vi "总磷总氮通讯.vi"() -> ()   [LabVIEW 2016, in "斯坦道总氮.lvlib"]
uses:
  <vilib>/NI/Modbus Library/API/Wrapper/Create TCP Slave.vi
  <vilib>/Utility/config.llb/Write Key (Boolean).vi
  <vilib>/Utility/config.llb/Write Key (String).vi
  <vilib>/Plasmionique/MB Master/MB_Master/MB_Master.lvclass
  <vilib>/NI/Modbus Library/API/Slave/Modbus Slave.lvclass
  <vilib>/Utility/config.llb/NI_LVConfig.lvlib
  <vilib>/Plasmionique/MB Master/MB Master.lvlib
  <vilib>/NI/Modbus Library/API/Wrapper/API Main.lvlib
panel:
  out "氨氮状态告警区":u16[](array[numeric])
  out "氨氮测量数据区":u16[](array[numeric])
  out "COD测量数据区":u16[](array[numeric])
  out "COD状态告警区":u16[](array[numeric])
  out "总氮测量数据区":u16[](array[numeric])
  out "总氮状态告警区":u16[](array[numeric])
  out "总磷状态告警区":u16[](array[numeric])
  out "总磷测量数据区":u16[](array[numeric])
  out "序列号":string
  out "状态告警区":T1 {"告警代码" items=["无告警", "缺试剂告警", "缺水样告警", "缺蒸馏水告警", "缺标液告警", "仪表漏液告警", "标定异常告警", "超量程告警", "加热异常", "低试剂预警", "超上限告警", "超下限告警", "仪表内部其他异常", "滴定异常告警", "电极异常告警", "量程切换告警", "参数设置告警", "PH电极电位异常", "电导率电极异常", "浊度光度异常", "溶解氧电极异常", "溶解氧光强异常", "温度异常告警", "PH异常告警", "溶解氧异常告警", "电导率异常告警", "浊度异常告警", "叶绿素异常告警", "藻密度异常告警", "蓝绿藻异常告警", "ORP异常告警", "氨氮异常告警", "清洁刷异常告警", "SD卡异常告警", "蓝牙异常告警", "Wifi异常告警", "流程异常告警"]; "故障代码" items=["无故障", "电机故障", "温度故障", "通讯故障", "滴定故障"]}
  out "测量数据区":T2 {"单位" items=["ug/L", "mg/L", "ppm", "mg/m3", "cm", "ppb", "ug/m3", "%", "nmol/mol", "umol/mol", "MPN/L", "MPN/100ml", "ng/m3", "NTU", "无量纲", "ms/cm", "us/cm", "℃", "mV", "万个/L"]}
  out "status":bool
  out "关键参数区":T3
  in  "读关键参数区":bool
  in  "读状态告警区":bool
  in  "读测量数据区":bool
  in  "站号":u16(ring) items=["总磷"=1, "氨氮"=3]
  in  "停止":bool
  in  "启动":bool
  in  "控制命令":u16(ring) items=["启动测量"=1, "标样核查"=2, "零点核查"=3, "跨度核查"=4, "空白测试"=5, "平行样测试"=6, "加标回收"=7, "空白校准"=8, "标样校准"=9, "初始化（清洗）"=10, "停止测试"=11, "仪器重启"=12, "校时"=13, "模式设置"=14, "测量间隔设置"=15]
  in  "控制命令参数":u16[](array[numeric]) format="%04xH"
  in  "VISA Resource":refnum<visa-resource-name>
  in  "启用模块":bool
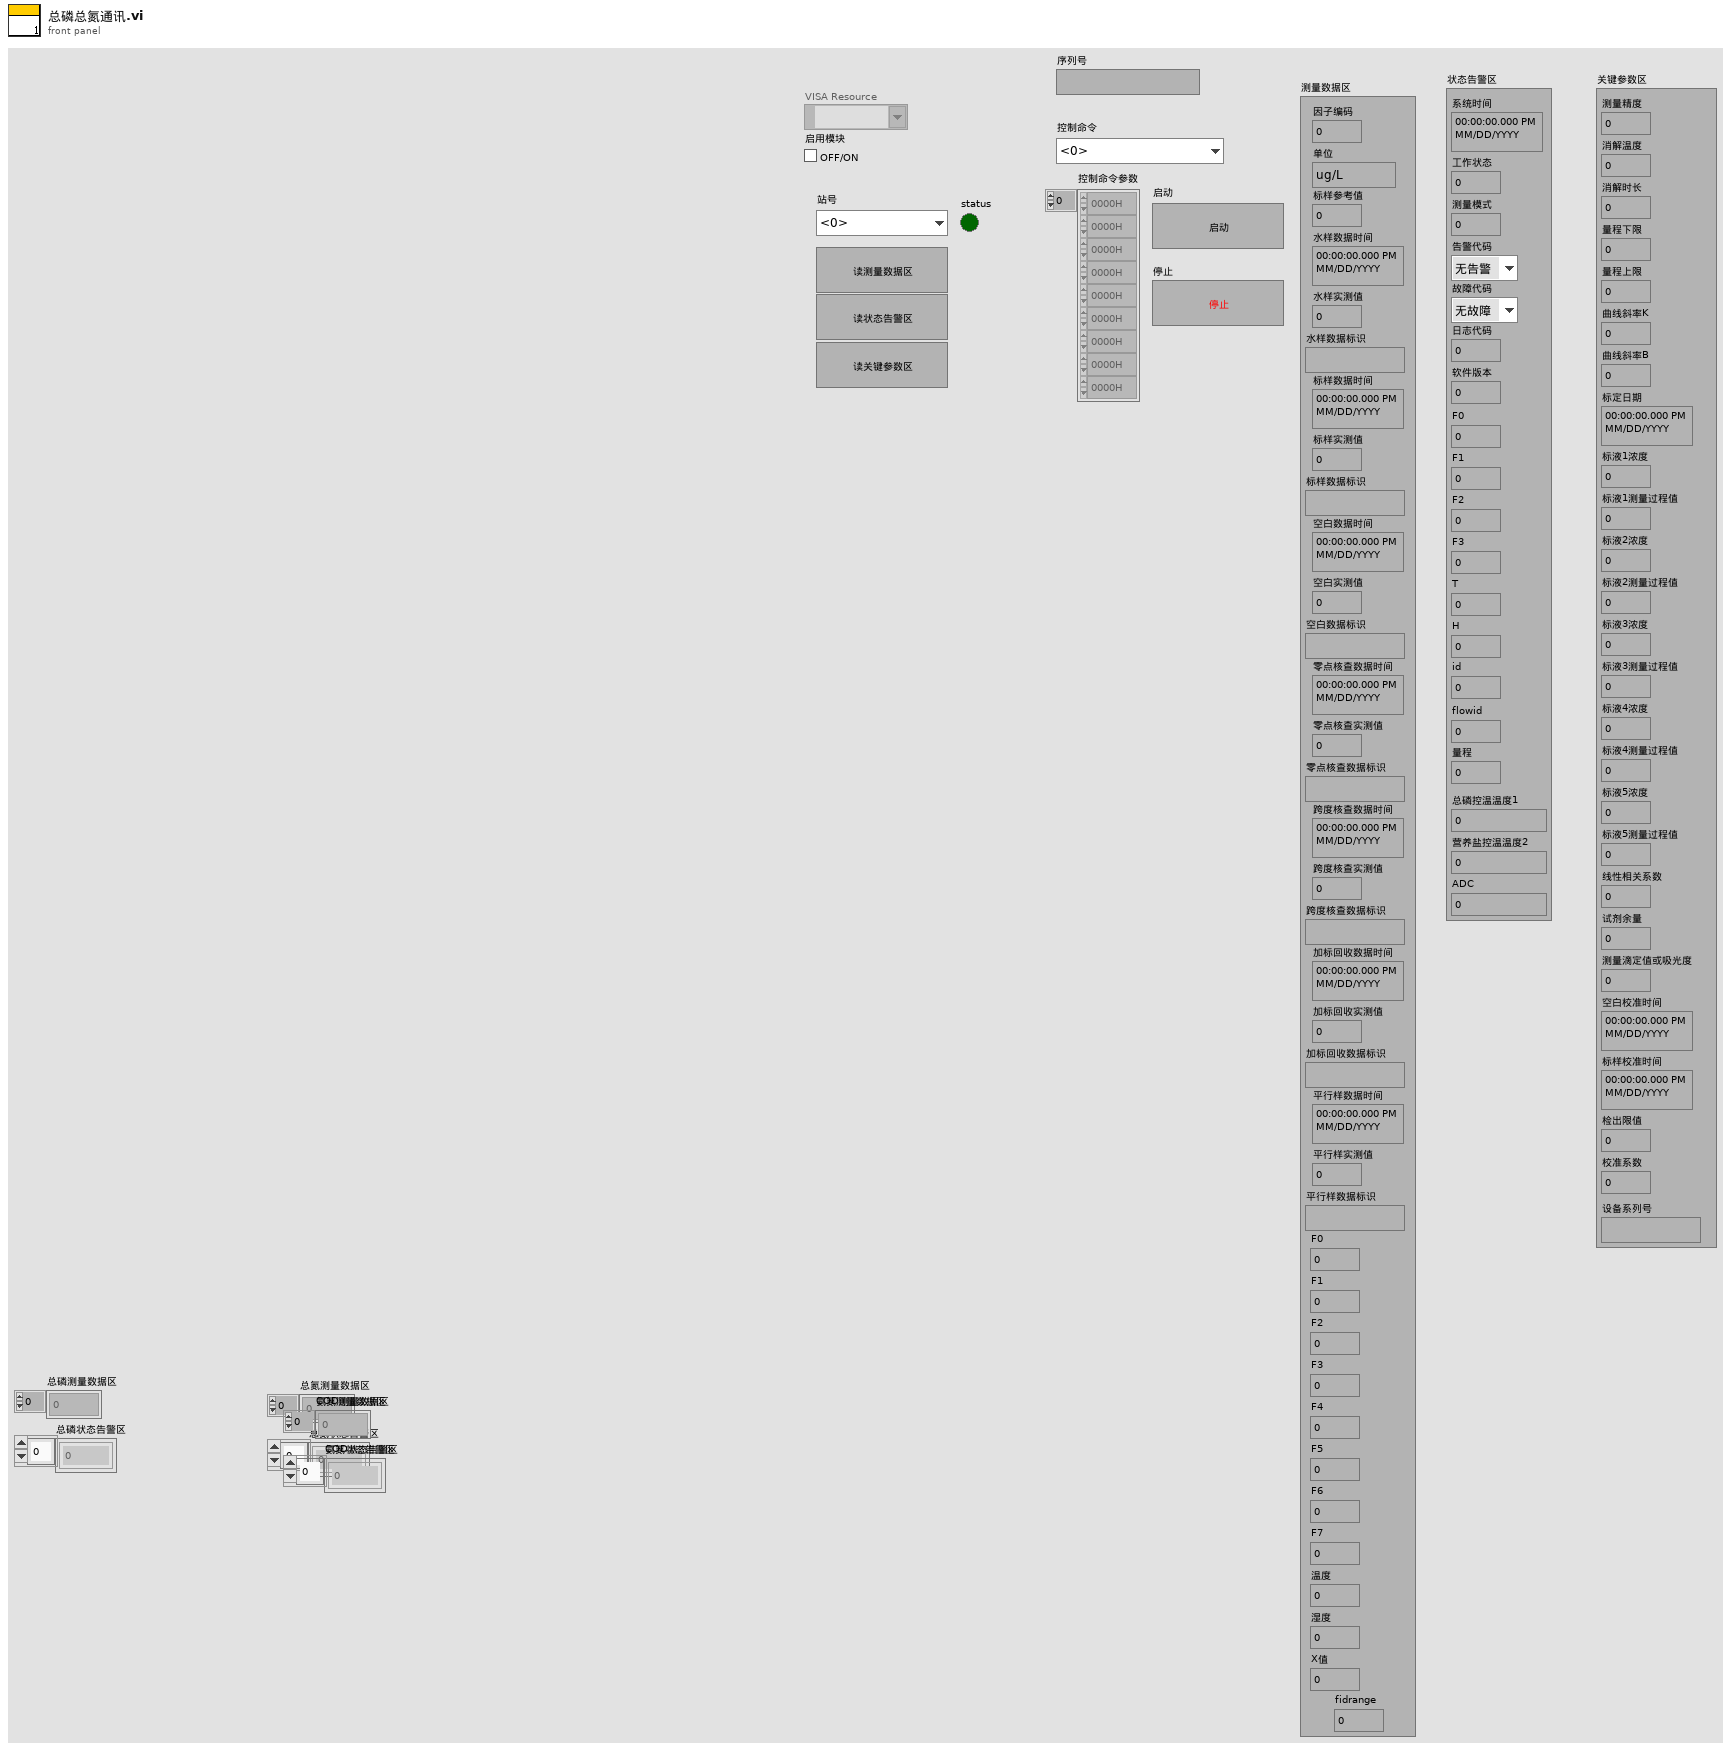
[diagram p1: front panel]
types:
  T1 = cluster{"系统时间":timestamp, "工作状态":u16, "测量模式":u16, "告警代码":u16, "故障代码":u16, "日志代码":u16, "软件版本":u16, "F0":sgl, "F1":sgl, "F2":sgl, "F3":sgl, "T":sgl, "H":sgl, "id":u16, "flowid":u16, "量程":u16, "总磷控温温度1":sgl, "营养盐控温温度2":sgl, "ADC":sgl}
  T2 = cluster{"因子编码":u32, "单位":u16, "标样参考值":sgl, "水样数据时间":timestamp, "水样实测值":sgl, "水样数据标识":string, "标样数据时间":timestamp, "标样实测值":sgl, "标样数据标识":string, "空白数据时间":timestamp, "空白实测值":sgl, "空白数据标识":string, "零点核查数据时间":timestamp, "零点核查实测值":sgl, "零点核查数据标识":string, "跨度核查数据时间":timestamp, "跨度核查实测值":sgl, "跨度核查数据标识":string, "加标回收数据时间":timestamp, "加标回收实测值":sgl, "加标回收数据标识":string, "平行样数据时间":timestamp, "平行样实测值":sgl, "平行样数据标识":string, "F0":sgl, "F1":sgl, "F2":sgl, "F3":sgl, "F4":sgl, "F5":sgl, "F6":sgl, "F7":sgl, "温度":sgl, "湿度":sgl, "X值":sgl, "fidrange":u16}
  T3 = cluster{"测量精度":u16, "消解温度":u16, "消解时长":u16, "量程下限":sgl, "量程上限":sgl, "曲线斜率K":sgl, "曲线斜率B":sgl, "标定日期":timestamp, "标液1浓度":sgl, "标液1测量过程值":sgl, "标液2浓度":sgl, "标液2测量过程值":sgl, "标液3浓度":sgl, "标液3测量过程值":sgl, "标液4浓度":sgl, "标液4测量过程值":sgl, "标液5浓度":sgl, "标液5测量过程值":sgl, "线性相关系数":sgl, "试剂余量":u32, "测量滴定值或吸光度":sgl, "空白校准时间":timestamp, "标样校准时间":timestamp, "检出限值":sgl, "校准系数":sgl, "设备系列号":string}
  T4 = cluster{"COD":bool, "氨氮":bool, "总氮":bool, "总磷":bool}
  T5 = typedef "NI_LVConfig.lvlib/Config Data RefNum.ctl" = refnum<k1>
  T6 = enum8{"Enabled", "Disabled", "Disabled and Grayed Out"}
  T7 = cluster{"系统时间":timestamp, "工作状态":enum16{"空闲", "水样测试", "标样核查", "零点核查", "跨度核查", "空白测试", "平行样测试", "加标回收", "空白校准", "标样校准", "初始化（清洗）"}, "测量模式":enum16{"待机", "连续模式", "周期模式", "定点模式", "受控模式", "手动模式"}, "告警代码":u16, "故障代码":u16, "日志代码":u16, "软件版本":u16, "F0":sgl, "F1":sgl, "F2":sgl, "F3":sgl, "T":sgl, "H":sgl, "id":u16, "flowid":u16, "量程":u16, "总磷控温温度1":sgl, "营养盐控温温度2":sgl, "ADC":sgl}
  T8 = cluster{"水样测试量程模式":enum16{"H", "L", "AUTO"}, "空白核查量程模式":enum16{"H", "L", "AUTO"}, "跨度核查量程模式":enum16{"H", "L", "AUTO"}, "加标回收量程模式":enum16{"H", "L", "AUTO"}}
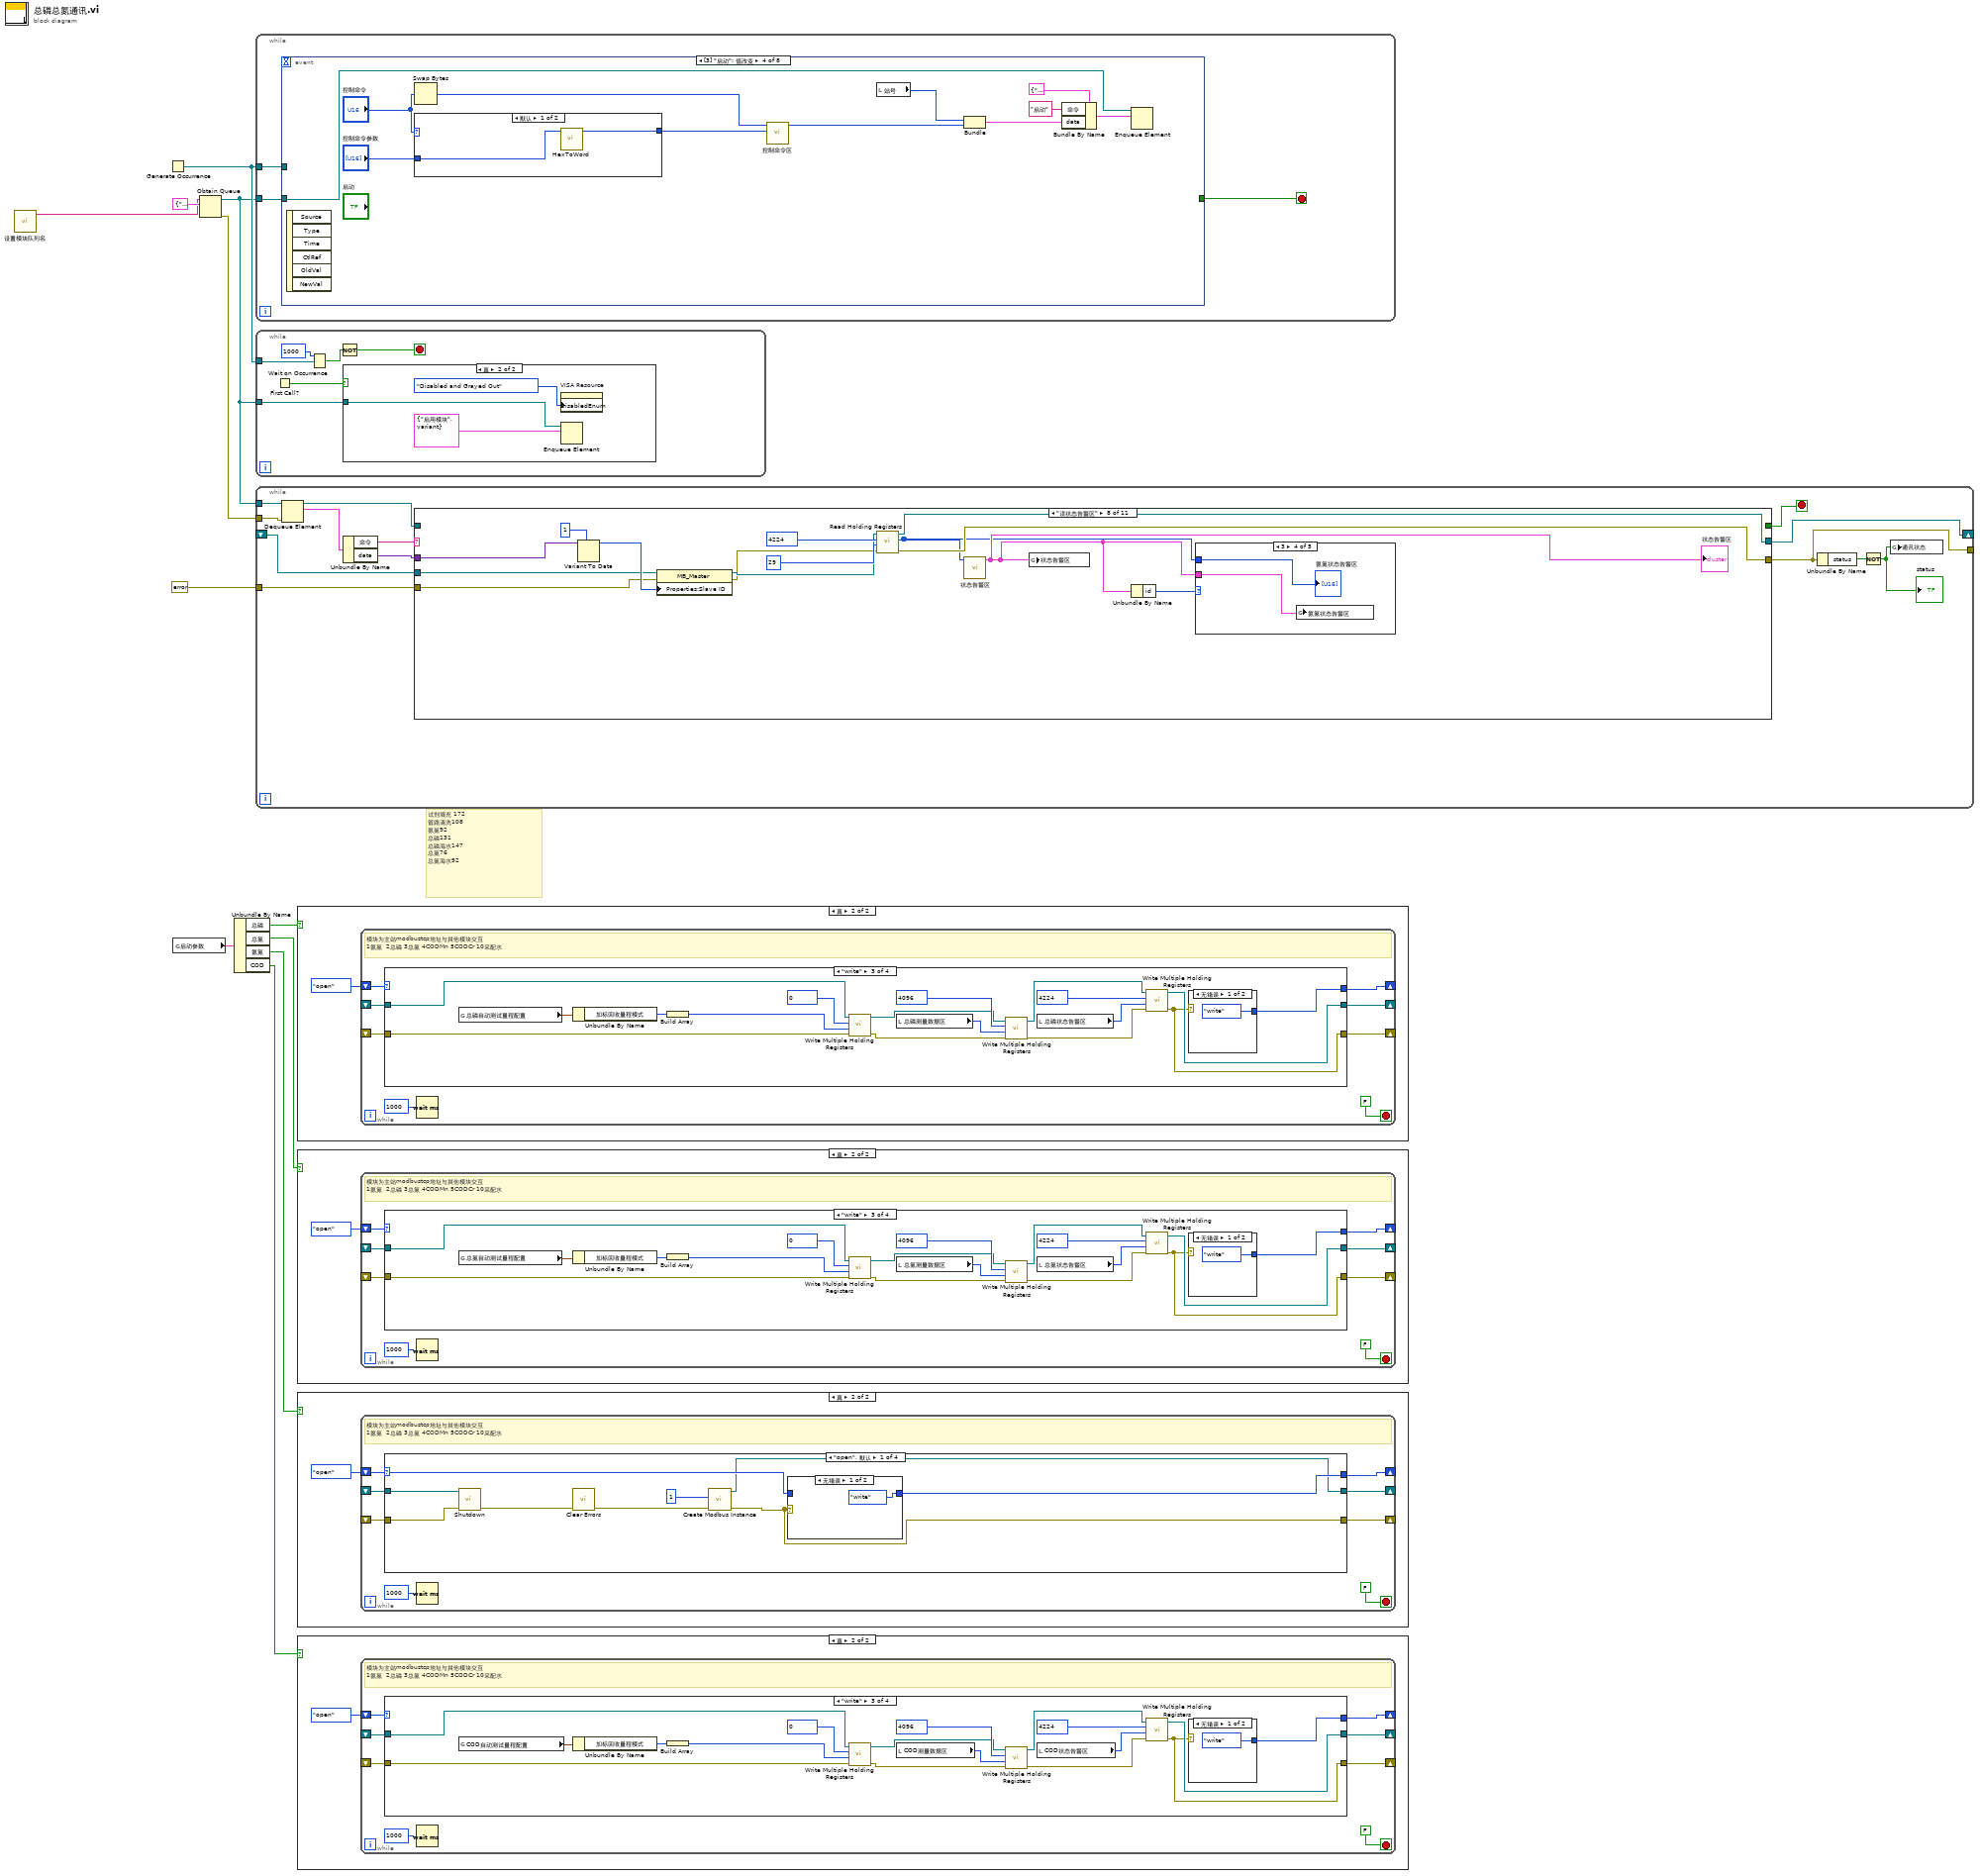
[diagram p0: block diagram]
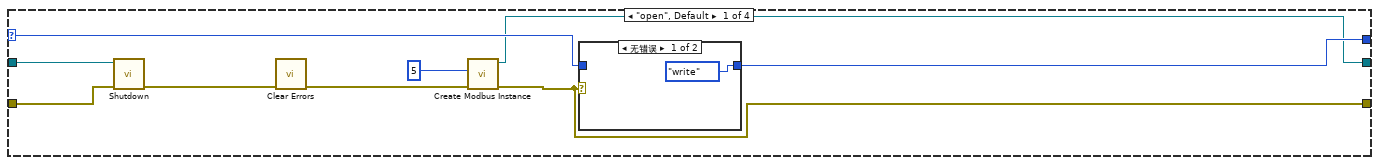
[diagram p3: hidden frame]
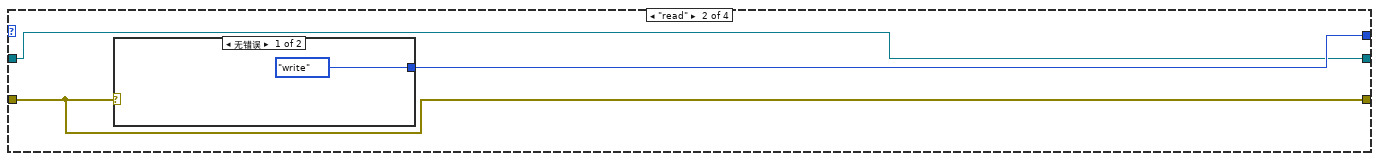
[diagram p5: hidden frame]
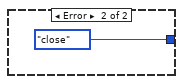
[diagram p6: hidden frame]
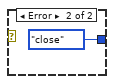
[diagram p7: hidden frame]
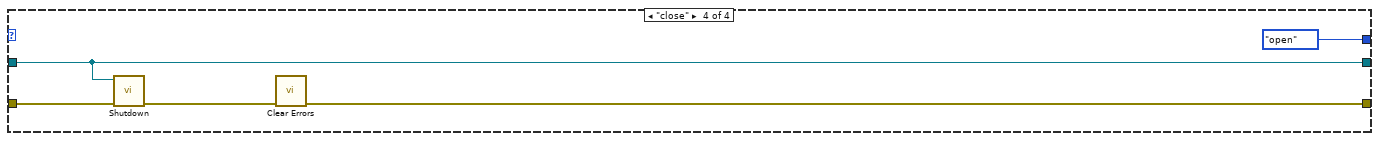
[diagram p8: hidden frame]
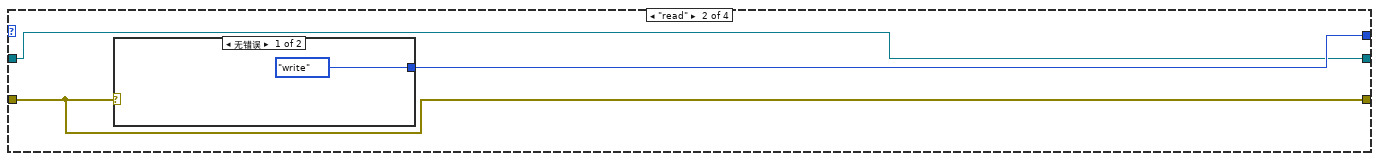
[diagram p11: hidden frame]
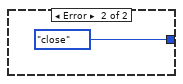
[diagram p12: hidden frame]
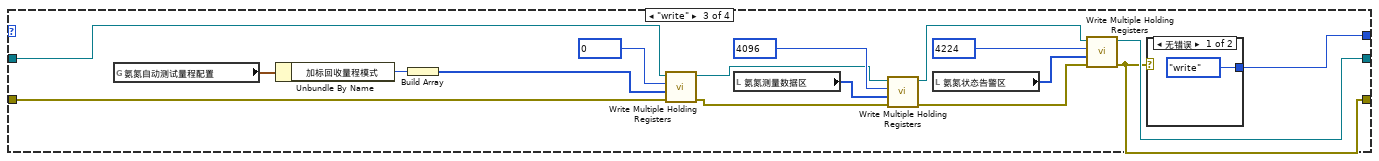
[diagram p13: hidden frame]
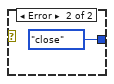
[diagram p14: hidden frame]
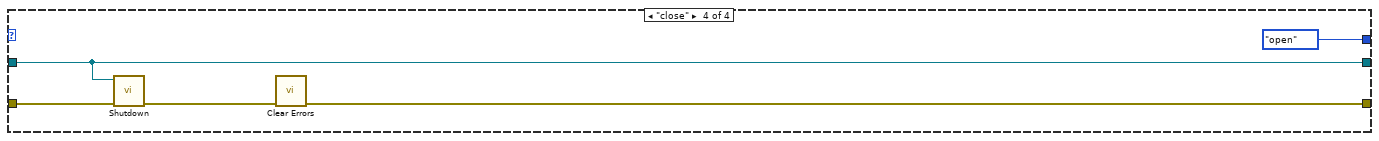
[diagram p15: hidden frame]
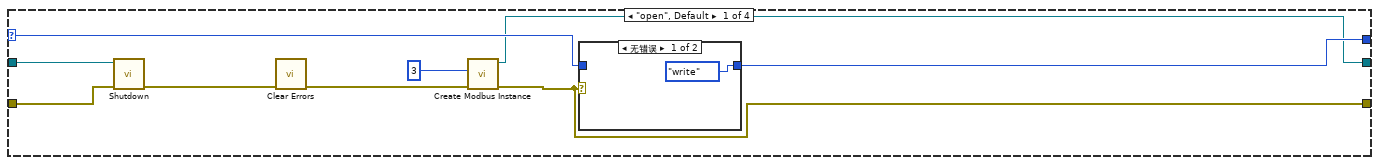
[diagram p17: hidden frame]
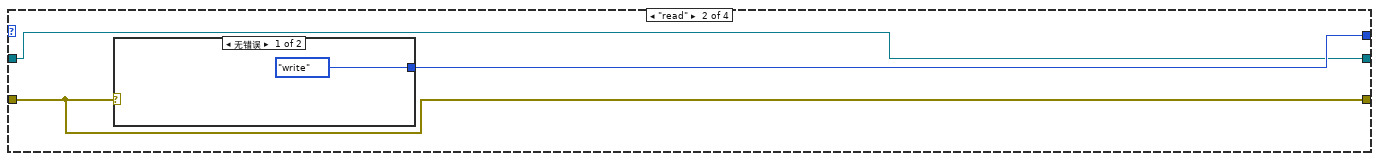
[diagram p19: hidden frame]
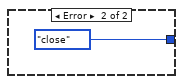
[diagram p20: hidden frame]
diagram:
  # "试剂填充 172 \n管路清洗108\n氨氮92\n总磷131\n总磷海水147\n总氮76\n总氮海水92"
  n1 = call "设置模块队列名.vi"() -> ("Msg"=w1:string)  [unwired: 5 in]
  n2 = Generate Occurrence() -> (w8:refnum<k4>)
  n3 = global read "总磷总氮断电保存全局变量.vi" "启动参数"() -> (w6:T4)
  n4 = Obtain Queue(name (unnamed)=w1, element data type=cluster{"命令":string, "data":variant} {"命令"="", "data"=variant}) -> (queue out=w7:refnum<queue>, error out=w10:errorcluster)  [unwired: 3 in, 1 out]
  n5 = Unbundle By Name(w6) -> ("总磷"=w5:bool, "总氮"=w4:bool, "氨氮"=w3:bool, "COD"=w2:bool)
  n6 = while {
    tunnel: w7 -> [w14]
    tunnel: w8 -> [w12]
    stop <- w13 stop-if-true
    n7 = event shown="[3] \"启动\": 值改变" {
      selector: _ -> [_ _ _ _ _ _ _ _]
      dyn-events: _ -> [_ _ _ _ _ _ _ _]
      timeout: _ -> [_ _ _ _ _ _ _ _]
      tunnel: w14 -> [_ _ _ w45 w52 w58 w63 w68]
      tunnel: [_ _ _ _ "停止" _ _ _] -> w13
      tunnel: w12 -> [_ _ _ _ w49 _ _ _]
      event Timeout {
        n8 = event-data() -> ()  [unwired: 1 in, 3 out]
      }
      event "启用模块": Value Change {
        n9 = event-data() -> ("NewVal"=w15:bool)  [unwired: 1 in, 5 out]
        n10 = call <vilib>:"Application Directory.vi"() -> ("Application Directory"=w17:path)
        n11 = Build Path(base path=w17, name or relative path="data\\set.ini" ("名称或相对路径")) -> (appended path=w18:path)
        n12 = call <vilib>:"Open Config Data.vi"("configuration file path"=w18) -> ("error out"=w24:errorcluster, "refnum"=w23:T5)  [unwired: 8 in, 1 out]
        n13 = call-poly <vilib>:"Write Key.vi"("section"="总磷总氮", "error in (no error)"=w24, "value"=w15, "key"="模块启用", "refnum"=w23) -> ("error out"=w20:errorcluster, "refnum out"=w16:T5)  [unwired: 4 in, 1 out]
        n14 = call <vilib>:"Close Config Data.vi"("error in (no error)"=w20, "refnum"=w16) -> ()  [unwired: 8 in, 2 out]
      }
      event "VISA Resource": Value Change {
        n15 = event-data() -> ()  [unwired: 1 in, 6 out]
        n16 = call <vilib>:"Application Directory.vi"() -> ("Application Directory"=w27:path)
        n17 = Build Path(base path=w27, name or relative path="data\\set.ini" ("名称或相对路径")) -> (appended path=w28:path)
        n18 = call <vilib>:"Open Config Data.vi"("configuration file path"=w28) -> ("error out"=w34:errorcluster, "refnum"=w33:T5)  [unwired: 8 in, 1 out]
        n19 = call-poly <vilib>:"Write Key.vi"("section"="总磷总氮", "error in (no error)"=w34, "value"="VISA Resource", "key"="串口", "refnum"=w33) -> ("error out"=w30:errorcluster, "refnum out"=w26:T5)  [unwired: 4 in, 1 out]
        n20 = call <vilib>:"Close Config Data.vi"("error in (no error)"=w30, "refnum"=w26) -> ()  [unwired: 8 in, 2 out]
      }
      event "启动": Value Change {
        n21 = event-data() -> ()  [unwired: 1 in, 6 out]
        n22 = Swap Bytes(anything="控制命令") -> (byte swapped=w38:u16)
        n23 = case shown="默认" "控制命令" {
          tunnel: "控制命令参数" -> [w47 w48]
          tunnel: [w46 w48] -> w35
          frame Default {
            n24 = call "HexToWord.vi"("数组"=w47) -> ("WORD"=w46:u16[])  [unwired: 10 in]
          }
          frame 13 {
          }
        }
        n25 = call "控制命令区.vi"("控制命令参数"=w35, "控制命令"=w38) -> ("控制命令"=w41:u16[])  [unwired: 9 in]
        n26 = local read "站号"() -> (w40:u16)
        n27 = Bundle("站号"=w40, "控制命令"=w41) -> (w39:cluster{"站号":u16, "控制命令":u16[]})  [unwired: 1 in]
        n28 = Bundle By Name(cluster=cluster{"命令":string, "data":variant} {"命令"="", "data"=variant} ("元素"), "命令"="启动", "data"=w39) -> (w43:cluster{"命令":string, "data":variant})
        n29 = Enqueue Element(queue=w45, element=w43) -> ()  [unwired: 2 in, 3 out]
      }
      event "停止": Value Change {
        n30 = event-data() -> ()  [unwired: 1 in, 6 out]
        n31 = Set Occurrence(w49) -> ()
        n32 = Flush Queue(queue=w52) -> (queue out=w51:refnum<queue>)  [unwired: 1 in, 2 out]
        n33 = Enqueue Element(queue=w51, element=cluster{"命令":string, "data":variant} {"命令"="shutdown", "data"=variant} ("元素")) -> ()  [unwired: 2 in, 3 out]
      }
      event "读测量数据区": Value Change {
        n34 = event-data() -> ()  [unwired: 1 in, 6 out]
        n35 = Bundle By Name(cluster=cluster{"命令":string, "data":variant} {"命令"="", "data"=variant} ("元素"), "命令"="读测量数据区", "data"="站号") -> (w56:cluster{"命令":string, "data":variant})
        n36 = Enqueue Element(queue=w58, element=w56) -> ()  [unwired: 2 in, 3 out]
      }
      event "读状态告警区": Value Change {
        n37 = event-data() -> ()  [unwired: 1 in, 6 out]
        n38 = local read "站号"() -> (w59:u16)
        n39 = Bundle By Name(cluster=cluster{"命令":string, "data":variant} {"命令"="", "data"=variant} ("元素"), "命令"="读状态告警区", "data"=w59) -> (w61:cluster{"命令":string, "data":variant})
        n40 = Enqueue Element(queue=w63, element=w61) -> ()  [unwired: 2 in, 3 out]
      }
      event "读关键参数区": Value Change {
        n41 = event-data() -> ()  [unwired: 1 in, 6 out]
        n42 = local read "站号"() -> (w64:u16)
        n43 = Bundle By Name(cluster=cluster{"命令":string, "data":variant} {"命令"="", "data"=variant} ("元素"), "命令"="读关键参数区", "data"=w64) -> (w66:cluster{"命令":string, "data":variant})
        n44 = Enqueue Element(queue=w68, element=w66) -> ()  [unwired: 2 in, 3 out]
      }
    }
  }
  n45 = while {
    tunnel: w8 -> [w74]
    tunnel: w7 -> [w70]
    stop <- w71 stop-if-true
    n46 = First Call?() -> (First Call?: T/F=w69:bool)
    n47 = Wait on Occurrence(2:w74, 3:1000 ("毫秒超时(-1)")) -> (0:w72:bool)  [unwired: 1 in]
    n48 = Not(x=w72) -> (.not. x?=w71:bool)
    n49 = case shown="真" w69 {
      tunnel: w70 -> [_ w76]
      frame False {
      }
      frame True {
        n50 = property on="VISA Resource" class="VISAName"("DisabledEnum"=T6."Disabled and Grayed Out" ("禁用")) -> ()  [unwired: 2 in, 2 out]
        n51 = Enqueue Element(queue=w76, element=cluster{"命令":string, "data":variant} {"命令"="启用模块", "data"=variant} ("元素")) -> ()  [unwired: 2 in, 3 out]
      }
    }
  }
  n52 = while {
    tunnel: w7 -> [w90]
    tunnel: w10 -> [w89]
    shift-right: [w87] -> _
    shift-left: _ -> [w86]
    tunnel: errorcluster {"status"=FALSE, "code"=0, "source"=""} ("error out") -> [w85]
    tunnel: [w80] -> _
    stop <- w88 stop-if-true
    n53 = Dequeue Element(queue=w90, error in (no error)=w89) -> (queue out=w81:refnum<queue>, element=w83:cluster{"命令":string, "data":variant})  [unwired: 1 in, 2 out]
    n54 = Unbundle By Name(w83) -> ("命令"=w84:string, "data"=w82:variant)
    n55 = case shown="\"读状态告警区\"" w84 {
      tunnel: w82 -> [_ _ _ w109 w120 w137 w147 w173 w195 w209 _]
      tunnel: w81 -> [_ _ _ _ _ _ _ _ _ _ w222]
      tunnel: [_ _ _ _ _ _ _ _ _ _ TRUE] -> w88
      tunnel: [w91 w93 w96 w112 w123 w139 w151 w182 w202 w216 w218] -> w87
      tunnel: [w92 w94 w97 w111 w122 w138 w152 w172 w203 w217 w219] -> w80
      tunnel: w86 -> [w91 _ w96 w108 w119 w136 w146 w176 w198 w212 w218]
      tunnel: w85 -> [w92 _ w99 w105 w116 w133 w144 w177 w199 w213 w220]
      frame Default {
      }
      frame "启用模块" {
        n56 = call "总磷总氮MB_api.vi"("STEP"=enum16{"open", "read", "write", "close"}."open") -> ("error out"=w94:errorcluster, "MB session out"=w93:refnum<class "MB_Master.lvclass">)  [unwired: 8 in, 1 out]
        n57 = global write "VAR总磷总氮全局变量.vi" "MB session in"(w93) -> ()
      }
      frame "停用模块" {
        n58 = call-dynamic "Close Session.vi"("error in (no error)"=w99, "MB session in"=w96) -> ("error out"=w98:errorcluster)  [unwired: 9 in]
        n59 = call <vilib>:"Clear Errors.vi"("error in (no error)"=w98) -> ("error out"=w97:errorcluster)  [unwired: 5 in, 1 out]
      }
      frame "启动" {
        n60 = Variant To Data(type=cluster{"站号":u16, "控制命令":u16[]} {"站号"=0, "控制命令"=[]} ("输出簇"), Variant=w109) -> (data=w103:cluster{"站号":u16, "控制命令":u16[]})  [unwired: 1 in, 1 out]
        n61 = Unbundle By Name(w103) -> ("站号"=w102:u16, "控制命令"=w100:u16[])
        n62 = Index Array(array=w100) -> (element=w101:u16)  [unwired: 1 in]
        n63 = property class="MB_Master"(reference=w108, error in=w105, "Properties:Slave ID"=w102) -> (reference out=w107:refnum<class "MB_Master.lvclass">, error out=w106:errorcluster)
        n64 = global write "VAR总磷总氮全局变量.vi" "控制命令"(w101) -> ()
        n65 = call <vilib>:"Write Multiple Registers.vi"("error in (no error)"=w106, "values"=w100, "starting address"=u16 4608, "MB session in"=w107) -> ("error out"=w111:errorcluster, "MB session out"=w112:refnum<class "MB_Master.lvclass">)  [unwired: 6 in]
      }
      frame "盲样测试" {
        n66 = Variant To Data(type=0, Variant=w120) -> (data=w113:i32)  [unwired: 1 in, 1 out]
        n67 = case shown="默认" w113 {
          tunnel: [u16[] [] ("values") u16[] [33539, 0] ("values") u16[] [23555, 0] ("values")] -> w115
          frame Default {
          }
          frame 1 {
            # "总磷盲样测试命令"
          }
          frame 3 {
            # "氨氮盲样测试"
          }
        }
        n68 = property class="MB_Master"(reference=w119, error in=w116, "Properties:Slave ID"=w113) -> (reference out=w118:refnum<class "MB_Master.lvclass">, error out=w117:errorcluster)
        n69 = call <vilib>:"Write Multiple Registers.vi"("error in (no error)"=w117, "values"=w115, "starting address"=u16 24592, "MB session in"=w118) -> ("error out"=w122:errorcluster, "MB session out"=w123:refnum<class "MB_Master.lvclass">)  [unwired: 6 in]
      }
      frame "debug" {
        n70 = Variant To Data(type=cluster{"站号":u16, "控制命令":u16[]} {"站号"=0, "控制命令"=[]} ("输出簇"), Variant=w137) -> (data=w131:cluster{"站号":u16, "控制命令":u16[]})  [unwired: 1 in, 1 out]
        n71 = Unbundle By Name(w131) -> ("站号"=w130:u16, "控制命令"=w128:u16[])
        n72 = Index Array(array=w128) -> (element=w129:u16)  [unwired: 1 in]
        n73 = property class="MB_Master"(reference=w136, error in=w133, "Properties:Slave ID"=w130) -> (reference out=w135:refnum<class "MB_Master.lvclass">, error out=w134:errorcluster)
        n74 = global write "VAR总磷总氮全局变量.vi" "控制命令"(w129) -> ()
        n75 = call <vilib>:"Write Multiple Registers.vi"("error in (no error)"=w134, "values"=w128, "starting address"=u16 24594, "MB session in"=w135) -> ("error out"=w138:errorcluster, "MB session out"=w139:refnum<class "MB_Master.lvclass">)  [unwired: 6 in]
      }
      frame "读测量数据区" {
        n76 = Variant To Data(type=u8 1 ("Slave ID"), Variant=w147) -> (data=w142:u8)  [unwired: 1 in, 1 out]
        n77 = property class="MB_Master"(reference=w146, error in=w144, "Properties:Slave ID"=w142) -> (reference out=w145:refnum<class "MB_Master.lvclass">, error out=w143:errorcluster)
        n78 = call <vilib>:"Read Holding Registers.vi"("error in (no error)"=w143, "quantity"=u16 105, "starting address"=u16 4096, "MB session in"=w145) -> ("error out"=w152:errorcluster, "Registers"=w140:u16[], "MB session out"=w151:refnum<class "MB_Master.lvclass">)  [unwired: 5 in]
        n79 = call "测量数据区.vi"("数组"=w140) -> ("测量数据区"=w141:T2)  [unwired: 10 in]
        "测量数据区" <- w141
        n80 = global write "VAR总磷总氮全局变量.vi" "测量数据区"(w141) -> ()
        n81 = case shown="3" w142 {
          tunnel: w141 -> [_ w155 w164 w166 w168]
          tunnel: w140 -> [_ w156 w163 w165 w167]
          frame 0, Default {
          }
          frame 1 {
            n82 = global read "总磷总氮断电保存全局变量.vi" "启动参数"() -> (w154:T4)
            n83 = Unbundle By Name(w154) -> ("总氮"=w153:bool)
            n84 = case shown="真" w153 {
              tunnel: [w158 w161] -> w157
              tunnel: w155 -> [w158 w159]
              frame False {
              }
              frame True {
                # "启动总氮时间自动对齐"
                n85 = global read "VAR总磷总氮全局变量.vi" "总氮测量数据区"() -> (w162:T2)
                n86 = global read "VAR总磷总氮全局变量.vi" "总磷测量数据区"() -> (w160:T2)
                n87 = call "总磷数据时间处理.vi"("总磷修正数据输入"=w160, "总氮原始数据"=w162, "总磷原始数据"=w159) -> ("总磷修正数据输出"=w161:T2)  [unwired: 8 in]
              }
            }
            n88 = global write "VAR总磷总氮全局变量.vi" "总磷测量数据区"(w157) -> ()
            "总磷测量数据区" <- w156
          }
          frame 2 {
            n89 = global write "VAR总磷总氮全局变量.vi" "总氮测量数据区"(w164) -> ()
            "总氮测量数据区" <- w163
          }
          frame 3 {
            n90 = global write "VAR总磷总氮全局变量.vi" "氨氮测量数据区"(w166) -> ()
            "氨氮测量数据区" <- w165
          }
          frame 22 {
            n91 = global write "VAR总磷总氮全局变量.vi" "COD测量数据区"(w168) -> ()
            "COD测量数据区" <- w167
          }
        }
      }
      frame "读状态告警区" {
        n92 = Variant To Data(type=u8 1 ("Slave ID"), Variant=w173) -> (data=w178:u8)  [unwired: 1 in, 1 out]
        n93 = property class="MB_Master"(reference=w176, error in=w177, "Properties:Slave ID"=w178) -> (reference out=w175:refnum<class "MB_Master.lvclass">, error out=w174:errorcluster)
        n94 = call <vilib>:"Read Holding Registers.vi"("error in (no error)"=w174, "quantity"=u16 29, "starting address"=u16 4224, "MB session in"=w175) -> ("error out"=w172:errorcluster, "Registers"=w169:u16[], "MB session out"=w182:refnum<class "MB_Master.lvclass">)  [unwired: 5 in]
        n95 = call "状态告警区.vi"("数组"=w169) -> ("状态告警区"=w170:T7)  [unwired: 10 in]
        "状态告警区" <- w170
        n96 = global write "VAR总磷总氮全局变量.vi" "状态告警区"(w170) -> ()
        n97 = Unbundle By Name(w170) -> ("id"=w171:u16)
        n98 = case shown="3" w171 {
          tunnel: w170 -> [_ w184 w186 w188 w190]
          tunnel: w169 -> [_ w183 w185 w187 w189]
          frame 0, Default {
          }
          frame 1, 131 {
            n99 = global write "VAR总磷总氮全局变量.vi" "总磷状态告警区"(w184) -> ()
            "总磷状态告警区" <- w183
          }
          frame 2, 76 {
            n100 = global write "VAR总磷总氮全局变量.vi" "总氮状态告警区"(w186) -> ()
            "总氮状态告警区" <- w185
          }
          frame 3 {
            n101 = global write "VAR总磷总氮全局变量.vi" "氨氮状态告警区"(w188) -> ()
            "氨氮状态告警区" <- w187
          }
          frame 22 {
            n102 = global write "VAR总磷总氮全局变量.vi" "COD状态告警区"(w190) -> ()
            "COD状态告警区" <- w189
          }
        }
      }
      frame "读关键参数区" {
        n103 = Variant To Data(type=u8 1 ("Slave ID"), Variant=w195) -> (data=w193:u8)  [unwired: 1 in, 1 out]
        n104 = property class="MB_Master"(reference=w198, error in=w199, "Properties:Slave ID"=w193) -> (reference out=w197:refnum<class "MB_Master.lvclass">, error out=w196:errorcluster)
        n105 = call <vilib>:"Read Holding Registers.vi"("error in (no error)"=w196, "quantity"=u16 19, "starting address"=u16 4256, "MB session in"=w197) -> ("error out"=w203:errorcluster, "Registers"=w192:u16[], "MB session out"=w202:refnum<class "MB_Master.lvclass">)  [unwired: 5 in]
        n106 = call "关键参数区.vi"("数组"=w192) -> ("关键参数区"=w191:T3)  [unwired: 10 in]
        "关键参数区" <- w191
        n107 = global write "VAR总磷总氮全局变量.vi" "关键参数区"(w191) -> ()
      }
      frame "读序列号" {
        n108 = Variant To Data(type=u8 1 ("Slave ID"), Variant=w209) -> (data=w207:u8)  [unwired: 1 in, 1 out]
        n109 = property class="MB_Master"(reference=w212, error in=w213, "Properties:Slave ID"=w207) -> (reference out=w211:refnum<class "MB_Master.lvclass">, error out=w210:errorcluster)
        n110 = call <vilib>:"Read Holding Registers.vi"("error in (no error)"=w210, "quantity"=u16 6, "starting address"=u16 4, "MB session in"=w211) -> ("error out"=w217:errorcluster, "Registers"=w206:u16[], "MB session out"=w216:refnum<class "MB_Master.lvclass">)  [unwired: 5 in]
        n111 = call "HexToString.vi"("数组"=w206) -> ("STRING"=w205:string[])  [unwired: 10 in]
        n112 = Index Array(array=w205) -> (element=w204:string)  [unwired: 1 in]
        "序列号" <- w204
        n113 = global write "VAR总磷总氮全局变量.vi" "序列号"(w204) -> ()
      }
      frame "shutdown" {
        n114 = Flush Queue(queue=w222) -> (queue out=w221:refnum<queue>)  [unwired: 1 in, 2 out]
        n115 = call-dynamic "Close Session.vi"("error in (no error)"=w220, "MB session in"=w218) -> ("error out"=w219:errorcluster)  [unwired: 9 in]
        n116 = Release Queue(queue=w221) -> ()  [unwired: 2 in, 3 out]
      }
    }
    n117 = Unbundle By Name(w80) -> ("status"=w79:bool)
    n118 = Not(x=w79) -> (.not. x?=w78:bool)
    "status" <- w78
    n119 = global write "VAR总磷总氮全局变量.vi" "通讯状态"(w78) -> ()
  }
  n120 = case shown="真" w5 {
    frame False {
    }
    frame True {
      n121 = while {
        shift-right: [w230] -> _
        shift-left: _ -> [w232]
        shift-right: [w229] -> _
        shift-left: _ -> [w231]
        shift-right: [w226] -> _
        shift-left: enum16{"open", "read", "write", "close"}."open" -> [w227]
        stop <- FALSE stop-if-true
        # "模块为主站modbustcp地址与其他模块交互\n1氨氮  2总磷 3总氮 4CODMn 5CODCr 10采配水"
        n122 = case shown="\"write\"" w227 {
          selector: w227 -> [w241 _ _ _]
          tunnel: w232 -> [w235 w244 w255 w270]
          tunnel: w231 -> [w234 w245 w251 w269]
          tunnel: [w238 w244 w261 w270] -> w230
          tunnel: [w237 w245 w260 w272] -> w229
          tunnel: [w240 w246 w265 enum16{"open", "read", "write", "close"}."open"] -> w226
          frame "open", Default {
            n123 = call-dynamic "Shutdown.vi"("error in"=w234, "Modbus slave in"=w235) -> ("error out"=w233:errorcluster)  [unwired: 9 in]
            n124 = call <vilib>:"Clear Errors.vi"("error in (no error)"=w233) -> ("error out"=w236:errorcluster)  [unwired: 5 in, 1 out]
            n125 = call-poly <vilib>:"Create Modbus Instance.vi"("error in"=w236, "port (502)"=u16 2) -> ("error out"=w237:errorcluster, "TCP slave instance"=w238:refnum<class "Modbus Slave.lvclass">)  [unwired: 8 in]
            n126 = case shown="无错误" w237 {
              tunnel: w241 -> [_ w243]
              tunnel: [enum16{"open", "read", "write", "close"}."write" w243] -> w240
              frame No Error {
              }
              frame Error {
              }
            }
          }
          frame "read" {
            n127 = case shown="无错误" w245 {
              tunnel: [enum16{"open", "read", "write", "close"}."write" enum16{"open", "read", "write", "close"}."close"] -> w246
              frame No Error {
              }
              frame Error {
              }
            }
          }
          frame "write" {
            n128 = global read "总磷总氮断电保存全局变量.vi" "总磷自动测试量程配置"() -> (w254:T8)
            n129 = Unbundle By Name(w254) -> ("加标回收量程模式"=w253:enum16{"H", "L", "AUTO"})
            n130 = Build Array(w253) -> (w252:enum16{"H", "L", "AUTO"}[])
            n131 = call-dynamic "Write Multiple Holding Registers.vi"("error in"=w251, "registers to write"=w252, "starting address"=u16 0, "Modbus slave in"=w255) -> ("error out"=w249:errorcluster, "Modbus slave out"=w250:refnum<class "Modbus Slave.lvclass">)  [unwired: 6 in]
            n132 = local read "总磷测量数据区"() -> (w259:u16[])
            n133 = call-dynamic "Write Multiple Holding Registers.vi"("error in"=w249, "registers to write"=w259, "starting address"=u16 4096, "Modbus slave in"=w250) -> ("error out"=w262:errorcluster, "Modbus slave out"=w263:refnum<class "Modbus Slave.lvclass">)  [unwired: 6 in]
            n134 = local read "总磷状态告警区"() -> (w257:u16[])
            n135 = call-dynamic "Write Multiple Holding Registers.vi"("error in"=w262, "registers to write"=w257, "starting address"=u16 4224, "Modbus slave in"=w263) -> ("error out"=w260:errorcluster, "Modbus slave out"=w261:refnum<class "Modbus Slave.lvclass">)  [unwired: 6 in]
            n136 = case shown="无错误" w260 {
              tunnel: [enum16{"open", "read", "write", "close"}."write" enum16{"open", "read", "write", "close"}."close"] -> w265
              frame No Error {
              }
              frame Error {
              }
            }
          }
          frame "close" {
            n137 = call-dynamic "Shutdown.vi"("error in"=w269, "Modbus slave in"=w270) -> ("error out"=w268:errorcluster)  [unwired: 9 in]
            n138 = call <vilib>:"Clear Errors.vi"("error in (no error)"=w268) -> ("error out"=w272:errorcluster)  [unwired: 5 in, 1 out]
          }
        }
        n139 = Wait (ms)(milliseconds to wait=u32 1000 ("等待时间（毫秒）")) -> ()  [unwired: 1 out]
      }
    }
  }
  n140 = case shown="真" w4 {
    frame False {
    }
    frame True {
      n141 = while {
        shift-right: [w279] -> _
        shift-left: _ -> [w281]
        shift-right: [w278] -> _
        shift-left: _ -> [w280]
        shift-right: [w275] -> _
        shift-left: enum16{"open", "read", "write", "close"}."open" -> [w276]
        stop <- FALSE stop-if-true
        # "模块为主站modbustcp地址与其他模块交互\n1氨氮  2总磷 3总氮 4CODMn 5CODCr 10采配水"
        n142 = case shown="\"write\"" w276 {
          selector: w276 -> [w290 _ _ _]
          tunnel: w281 -> [w284 w293 w301 w319]
          tunnel: w280 -> [w283 w294 w300 w318]
          tunnel: [w287 w293 w310 w319] -> w279
          tunnel: [w286 w294 w309 w321] -> w278
          tunnel: [w289 w295 w314 enum16{"open", "read", "write", "close"}."open"] -> w275
          frame "open", Default {
            n143 = call-dynamic "Shutdown.vi"("error in"=w283, "Modbus slave in"=w284) -> ("error out"=w282:errorcluster)  [unwired: 9 in]
            n144 = call <vilib>:"Clear Errors.vi"("error in (no error)"=w282) -> ("error out"=w285:errorcluster)  [unwired: 5 in, 1 out]
            n145 = call-poly <vilib>:"Create Modbus Instance.vi"("error in"=w285, "port (502)"=u16 3) -> ("error out"=w286:errorcluster, "TCP slave instance"=w287:refnum<class "Modbus Slave.lvclass">)  [unwired: 8 in]
            n146 = case shown="无错误" w286 {
              tunnel: w290 -> [_ w292]
              tunnel: [enum16{"open", "read", "write", "close"}."write" w292] -> w289
              frame No Error {
              }
              frame Error {
              }
            }
          }
          frame "read" {
            n147 = case shown="无错误" w294 {
              tunnel: [enum16{"open", "read", "write", "close"}."write" enum16{"open", "read", "write", "close"}."close"] -> w295
              frame No Error {
              }
              frame Error {
              }
            }
          }
          frame "write" {
            n148 = global read "总磷总氮断电保存全局变量.vi" "总氮自动测试量程配置"() -> (w304:T8)
            n149 = Unbundle By Name(w304) -> ("加标回收量程模式"=w303:enum16{"H", "L", "AUTO"})
            n150 = Build Array(w303) -> (w302:enum16{"H", "L", "AUTO"}[])
            n151 = call-dynamic "Write Multiple Holding Registers.vi"("error in"=w300, "registers to write"=w302, "starting address"=u16 0, "Modbus slave in"=w301) -> ("error out"=w298:errorcluster, "Modbus slave out"=w299:refnum<class "Modbus Slave.lvclass">)  [unwired: 6 in]
            n152 = local read "总氮测量数据区"() -> (w308:u16[])
            n153 = call-dynamic "Write Multiple Holding Registers.vi"("error in"=w298, "registers to write"=w308, "starting address"=u16 4096, "Modbus slave in"=w299) -> ("error out"=w311:errorcluster, "Modbus slave out"=w312:refnum<class "Modbus Slave.lvclass">)  [unwired: 6 in]
            n154 = local read "总氮状态告警区"() -> (w306:u16[])
            n155 = call-dynamic "Write Multiple Holding Registers.vi"("error in"=w311, "registers to write"=w306, "starting address"=u16 4224, "Modbus slave in"=w312) -> ("error out"=w309:errorcluster, "Modbus slave out"=w310:refnum<class "Modbus Slave.lvclass">)  [unwired: 6 in]
            n156 = case shown="无错误" w309 {
              tunnel: [enum16{"open", "read", "write", "close"}."write" enum16{"open", "read", "write", "close"}."close"] -> w314
              frame No Error {
              }
              frame Error {
              }
            }
          }
          frame "close" {
            n157 = call-dynamic "Shutdown.vi"("error in"=w318, "Modbus slave in"=w319) -> ("error out"=w317:errorcluster)  [unwired: 9 in]
            n158 = call <vilib>:"Clear Errors.vi"("error in (no error)"=w317) -> ("error out"=w321:errorcluster)  [unwired: 5 in, 1 out]
          }
        }
        n159 = Wait (ms)(milliseconds to wait=u32 1000 ("等待时间（毫秒）")) -> ()  [unwired: 1 out]
      }
    }
  }
  n160 = case shown="真" w3 {
    frame False {
    }
    frame True {
      n161 = while {
        shift-right: [w328] -> _
        shift-left: _ -> [w330]
        shift-right: [w327] -> _
        shift-left: _ -> [w329]
        shift-right: [w324] -> _
        shift-left: enum16{"open", "read", "write", "close"}."open" -> [w325]
        stop <- FALSE stop-if-true
        # "模块为主站modbustcp地址与其他模块交互\n1氨氮  2总磷 3总氮 4CODMn 5CODCr 10采配水"
        n162 = case shown="\"open\", 默认" w325 {
          selector: w325 -> [w339 _ _ _]
          tunnel: w330 -> [w333 w342 w350 w368]
          tunnel: w329 -> [w332 w343 w349 w367]
          tunnel: [w336 w342 w359 w368] -> w328
          tunnel: [w335 w343 w358 w370] -> w327
          tunnel: [w338 w344 w363 enum16{"open", "read", "write", "close"}."open"] -> w324
          frame "open", Default {
            n163 = call-dynamic "Shutdown.vi"("error in"=w332, "Modbus slave in"=w333) -> ("error out"=w331:errorcluster)  [unwired: 9 in]
            n164 = call <vilib>:"Clear Errors.vi"("error in (no error)"=w331) -> ("error out"=w334:errorcluster)  [unwired: 5 in, 1 out]
            n165 = call-poly <vilib>:"Create Modbus Instance.vi"("error in"=w334, "port (502)"=u16 1) -> ("error out"=w335:errorcluster, "TCP slave instance"=w336:refnum<class "Modbus Slave.lvclass">)  [unwired: 8 in]
            n166 = case shown="无错误" w335 {
              tunnel: w339 -> [_ w341]
              tunnel: [enum16{"open", "read", "write", "close"}."write" w341] -> w338
              frame No Error {
              }
              frame Error {
              }
            }
          }
          frame "read" {
            n167 = case shown="无错误" w343 {
              tunnel: [enum16{"open", "read", "write", "close"}."write" enum16{"open", "read", "write", "close"}."close"] -> w344
              frame No Error {
              }
              frame Error {
              }
            }
          }
          frame "write" {
            n168 = global read "总磷总氮断电保存全局变量.vi" "氨氮自动测试量程配置"() -> (w353:T8)
            n169 = Unbundle By Name(w353) -> ("加标回收量程模式"=w352:enum16{"H", "L", "AUTO"})
            n170 = Build Array(w352) -> (w351:enum16{"H", "L", "AUTO"}[])
            n171 = call-dynamic "Write Multiple Holding Registers.vi"("error in"=w349, "registers to write"=w351, "starting address"=u16 0, "Modbus slave in"=w350) -> ("error out"=w347:errorcluster, "Modbus slave out"=w348:refnum<class "Modbus Slave.lvclass">)  [unwired: 6 in]
            n172 = local read "氨氮测量数据区"() -> (w357:u16[])
            n173 = call-dynamic "Write Multiple Holding Registers.vi"("error in"=w347, "registers to write"=w357, "starting address"=u16 4096, "Modbus slave in"=w348) -> ("error out"=w360:errorcluster, "Modbus slave out"=w361:refnum<class "Modbus Slave.lvclass">)  [unwired: 6 in]
            n174 = local read "氨氮状态告警区"() -> (w355:u16[])
            n175 = call-dynamic "Write Multiple Holding Registers.vi"("error in"=w360, "registers to write"=w355, "starting address"=u16 4224, "Modbus slave in"=w361) -> ("error out"=w358:errorcluster, "Modbus slave out"=w359:refnum<class "Modbus Slave.lvclass">)  [unwired: 6 in]
            n176 = case shown="无错误" w358 {
              tunnel: [enum16{"open", "read", "write", "close"}."write" enum16{"open", "read", "write", "close"}."close"] -> w363
              frame No Error {
              }
              frame Error {
              }
            }
          }
          frame "close" {
            n177 = call-dynamic "Shutdown.vi"("error in"=w367, "Modbus slave in"=w368) -> ("error out"=w366:errorcluster)  [unwired: 9 in]
            n178 = call <vilib>:"Clear Errors.vi"("error in (no error)"=w366) -> ("error out"=w370:errorcluster)  [unwired: 5 in, 1 out]
          }
        }
        n179 = Wait (ms)(milliseconds to wait=u32 1000 ("等待时间（毫秒）")) -> ()  [unwired: 1 out]
      }
    }
  }
  n180 = case shown="真" w2 {
    frame False {
    }
    frame True {
      n181 = while {
        shift-right: [w377] -> _
        shift-left: _ -> [w379]
        shift-right: [w376] -> _
        shift-left: _ -> [w378]
        shift-right: [w373] -> _
        shift-left: enum16{"open", "read", "write", "close"}."open" -> [w374]
        stop <- FALSE stop-if-true
        # "模块为主站modbustcp地址与其他模块交互\n1氨氮  2总磷 3总氮 4CODMn 5CODCr 10采配水"
        n182 = case shown="\"write\"" w374 {
          selector: w374 -> [w388 _ _ _]
          tunnel: w379 -> [w382 w391 w399 w417]
          tunnel: w378 -> [w381 w392 w398 w416]
          tunnel: [w385 w391 w408 w417] -> w377
          tunnel: [w384 w392 w407 w419] -> w376
          tunnel: [w387 w393 w412 enum16{"open", "read", "write", "close"}."open"] -> w373
          frame "open", Default {
            n183 = call-dynamic "Shutdown.vi"("error in"=w381, "Modbus slave in"=w382) -> ("error out"=w380:errorcluster)  [unwired: 9 in]
            n184 = call <vilib>:"Clear Errors.vi"("error in (no error)"=w380) -> ("error out"=w383:errorcluster)  [unwired: 5 in, 1 out]
            n185 = call-poly <vilib>:"Create Modbus Instance.vi"("error in"=w383, "port (502)"=u16 5) -> ("error out"=w384:errorcluster, "TCP slave instance"=w385:refnum<class "Modbus Slave.lvclass">)  [unwired: 8 in]
            n186 = case shown="无错误" w384 {
              tunnel: w388 -> [_ w390]
              tunnel: [enum16{"open", "read", "write", "close"}."write" w390] -> w387
              frame No Error {
              }
              frame Error {
              }
            }
          }
          frame "read" {
            n187 = case shown="无错误" w392 {
              tunnel: [enum16{"open", "read", "write", "close"}."write" enum16{"open", "read", "write", "close"}."close"] -> w393
              frame No Error {
              }
              frame Error {
              }
            }
          }
          frame "write" {
            n188 = global read "总磷总氮断电保存全局变量.vi" "COD自动测试量程配置"() -> (w402:T8)
            n189 = Unbundle By Name(w402) -> ("加标回收量程模式"=w401:enum16{"H", "L", "AUTO"})
            n190 = Build Array(w401) -> (w400:enum16{"H", "L", "AUTO"}[])
            n191 = call-dynamic "Write Multiple Holding Registers.vi"("error in"=w398, "registers to write"=w400, "starting address"=u16 0, "Modbus slave in"=w399) -> ("error out"=w396:errorcluster, "Modbus slave out"=w397:refnum<class "Modbus Slave.lvclass">)  [unwired: 6 in]
            n192 = local read "COD测量数据区"() -> (w406:u16[])
            n193 = call-dynamic "Write Multiple Holding Registers.vi"("error in"=w396, "registers to write"=w406, "starting address"=u16 4096, "Modbus slave in"=w397) -> ("error out"=w409:errorcluster, "Modbus slave out"=w410:refnum<class "Modbus Slave.lvclass">)  [unwired: 6 in]
            n194 = local read "COD状态告警区"() -> (w404:u16[])
            n195 = call-dynamic "Write Multiple Holding Registers.vi"("error in"=w409, "registers to write"=w404, "starting address"=u16 4224, "Modbus slave in"=w410) -> ("error out"=w407:errorcluster, "Modbus slave out"=w408:refnum<class "Modbus Slave.lvclass">)  [unwired: 6 in]
            n196 = case shown="无错误" w407 {
              tunnel: [enum16{"open", "read", "write", "close"}."write" enum16{"open", "read", "write", "close"}."close"] -> w412
              frame No Error {
              }
              frame Error {
              }
            }
          }
          frame "close" {
            n197 = call-dynamic "Shutdown.vi"("error in"=w416, "Modbus slave in"=w417) -> ("error out"=w415:errorcluster)  [unwired: 9 in]
            n198 = call <vilib>:"Clear Errors.vi"("error in (no error)"=w415) -> ("error out"=w419:errorcluster)  [unwired: 5 in, 1 out]
          }
        }
        n199 = Wait (ms)(milliseconds to wait=u32 1000 ("等待时间（毫秒）")) -> ()  [unwired: 1 out]
      }
    }
  }
